vi "Line_Notify_test.vi"() -> ()   [LabVIEW 2019]
panel:
  in  "String":string
  in  "Send message":bool
  in  "stop":bool
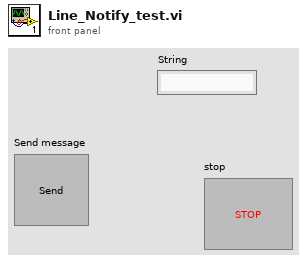
[diagram p1: front panel]
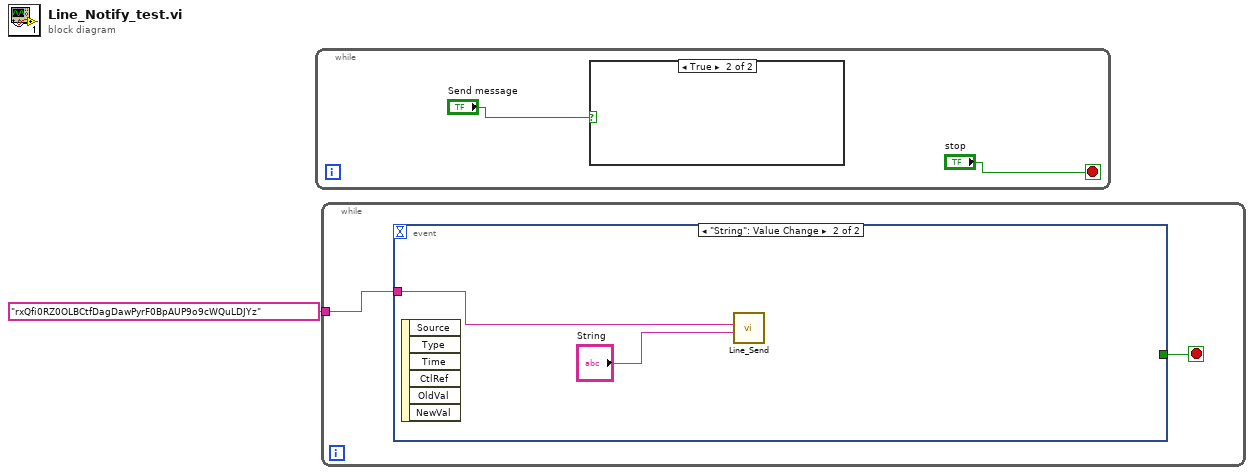
[diagram p0: block diagram]
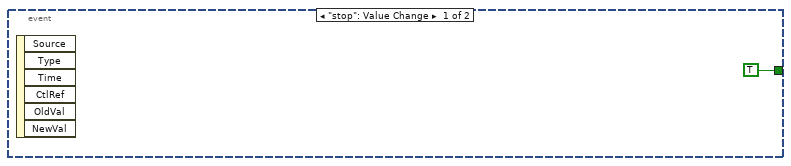
[diagram p3: hidden frame]
diagram:
  n1 = while {
    stop <- "stop" stop-if-true
    n2 = case shown="True" "Send message" {
      frame False {
      }
      frame True {
      }
    }
  }
  n3 = while {
    tunnel: "rxQfi0RZ0OLBCtfDagDawPyrF0BpAUP9o9cWQuLDJYz" -> [w4]
    stop <- w5 stop-if-true
    n4 = event shown="[1] \"String\": Value Change" {
      selector: _ -> [_ _]
      dyn-events: _ -> [_ _]
      timeout: _ -> [_ _]
      tunnel: [TRUE _] -> w5
      tunnel: w4 -> [_ w8]
      event "stop": Value Change {
        n5 = event-data() -> ()  [unwired: 1 in, 6 out]
      }
      event "String": Value Change {
        n6 = event-data() -> ()  [unwired: 1 in, 6 out]
        n7 = call "Line_Send.vi"("message"="String", "Key"=w8) -> ()  [unwired: 10 in]
      }
    }
  }
